vi "Buffer Initialize.vi"(8 "error in (no error)":errorcluster, 9 "Number Of Elements":i32[](array[numeric]), 10 "Sector Number":i32, 11 "Circular Buffer 2D U16 DVR Queue Circular Buffer in":refnum<class "Circular Buffer 2D U16 DVR Queue Circular Buffer.lvclass">) -> (0 "error out":errorcluster, 3 "Circular Buffer 2D U16 DVR Queue Circular Buffer out":refnum<class "Circular Buffer 2D U16 DVR Queue Circular Buffer.lvclass">)   [LabVIEW 2024, in "Circular Buffer 2D U16 DVR Queue Circular Buffer.lvclass"]
uses:
  Circular Buffer 2D U16 DVR Queue Circular Buffer.lvclass
  Type Def/2D U16 DVR.ctl
  Circular Buffer 2D U16 DVR Queue Circular Buffer.lvclass/Circular Buffer 2D U16 DVR Queue Circular Buffer.ctl
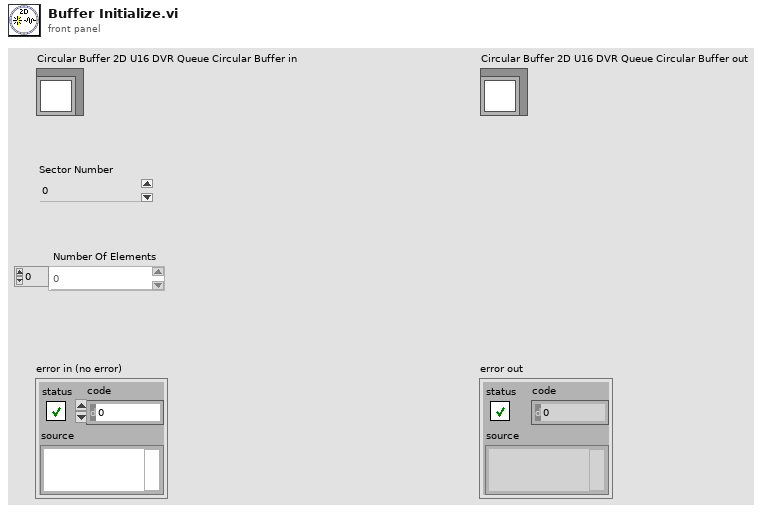
[diagram p1: front panel]
types:
  T1 = typedef "2D U16 DVR.ctl" = refnum<data-value>
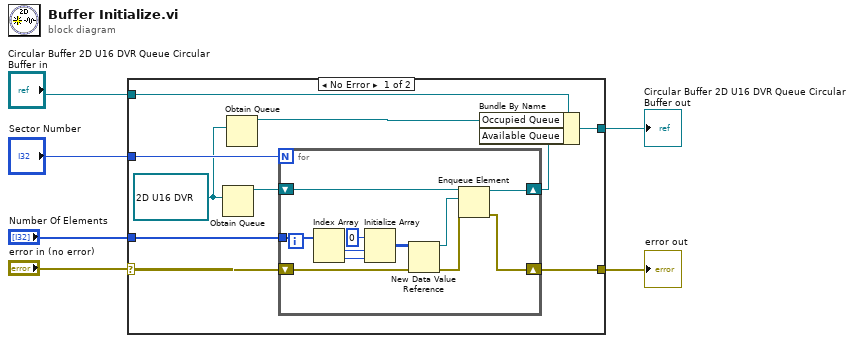
[diagram p0: block diagram]
diagram:
  n1 = case shown="No Error" "error in (no error)" {
    selector: "error in (no error)" -> [w16 w29]
    tunnel: [w15 w29] -> w5
    tunnel: "Sector Number" -> [w14 _]
    tunnel: "Number Of Elements" -> [w13 _]
    tunnel: "Circular Buffer 2D U16 DVR Queue Circular Buffer in" -> [w10 w28]
    tunnel: [w7 w28] -> w1
    frame No Error {
      w12 = T1 refnum ("2D U16 DVR")
      n2 = Obtain Queue(element data type=w12) -> (queue out=w11:refnum<queue>)  [unwired: 4 in, 2 out]
      n3 = Obtain Queue(element data type=w12) -> (queue out=w8:refnum<queue>)  [unwired: 4 in, 2 out]
      n4 = for {
        N: w14 -> [_]
        shift-right: [w17] -> w15
        shift-left: w16 -> [w22]
        tunnel: w13 -> [w27]
        shift-right: [w19] -> w9
        shift-left: w11 -> [w21]
        n5 = Index Array(array=w27) -> (element #1=w26:i32, element #2=w25:i32)  [unwired: 2 in]
        n6 = Initialize Array(u16 0 ("element"), w26, w25) -> (w23:u16[][])
        n7 = New Data Value Reference(data value=w23, error in=w22) -> (data value reference=w20:refnum<data-value>, error out=w18:errorcluster)
        n8 = Enqueue Element(queue=w21, element=w20, error in (no error)=w18) -> (queue out=w19:refnum<queue>, error out=w17:errorcluster)  [unwired: 1 in, 1 out]
      }
      n9 = Bundle By Name(cluster=w10, "Occupied Queue"=w8, "Available Queue"=w9) -> (w7:refnum<class "Circular Buffer 2D U16 DVR Queue Circular Buffer.lvclass">)
    }
    frame Error {
    }
  }
  "error out" <- w5
  "Circular Buffer 2D U16 DVR Queue Circular Buffer out" <- w1
